vi "Shut_Down_A_Tunnel.vi"(3 "Mode":T5=enum."Run VI", 5 "Traverse line In":T2 {"Carrier_2 Q (l/min)" format="%#.2f"; "Row Duration (mins)" format="%#.1f"; "Row No" min=0; "Trace Gas Concentration (%)" min=0.0 format="%#_4f"; "Carrier_1 Q (l/min)" format="%#.4f"; "Start X" format="%#.2f"; "Start Y" format="%#.2f"; "Start Z" format="%#.2f"; "End X" format="%#.2f"; "End Y" format="%#.2f"; "End Z" format="%#.2f"; "Tunnel Speed" format="%#.2f"; "Averaging time (mins)" min=0.0 format="%#.2f"}) -> (0 "Error Message":string, 1 "Status":T1, 2 "Traverse line Out":T2 {"Carrier_2 Q (l/min)" format="%#.2f"; "Row Duration (mins)" format="%#.1f"; "Row No" min=0; "Trace Gas Concentration (%)" min=0.0 format="%#_4f"; "Carrier_1 Q (l/min)" format="%#.4f"; "Start X" format="%#.2f"; "Start Y" format="%#.2f"; "Start Z" format="%#.2f"; "End X" format="%#.2f"; "End Y" format="%#.2f"; "End Z" format="%#.2f"; "Tunnel Speed" format="%#.2f"; "Averaging time (mins)" min=0.0 format="%#.2f"})   [LabVIEW 2022 SP3]
uses:
  Gen Trav/Traverse_cluster.ctl
  Gen Trav/Spacing.ctl
  Controls/Multi_run_mode.ctl
  Controls/User_Specific_mode.ctl
  Gen Trav/Multi_Run_Status.ctl
  Controls/GMU Gas Line Name.ctl
  ADAM Client/Sub VIs/ADAM Controls/Channel_names.ctl
  ADAM Client/Sub VIs/ADAM Controls/Client_Source_Status.ctl
  ADAM Client/Sub VIs/ADAM Controls/Tunnel_speed_mode.ctl
  Globals/Trav_pos_global.vi
  Globals/Preference_global.vi
panel:
  # "X           Y          Z"
  # "Start"
  # "End"
  # "X           Y          Z"
  # "Start"
  # "End"
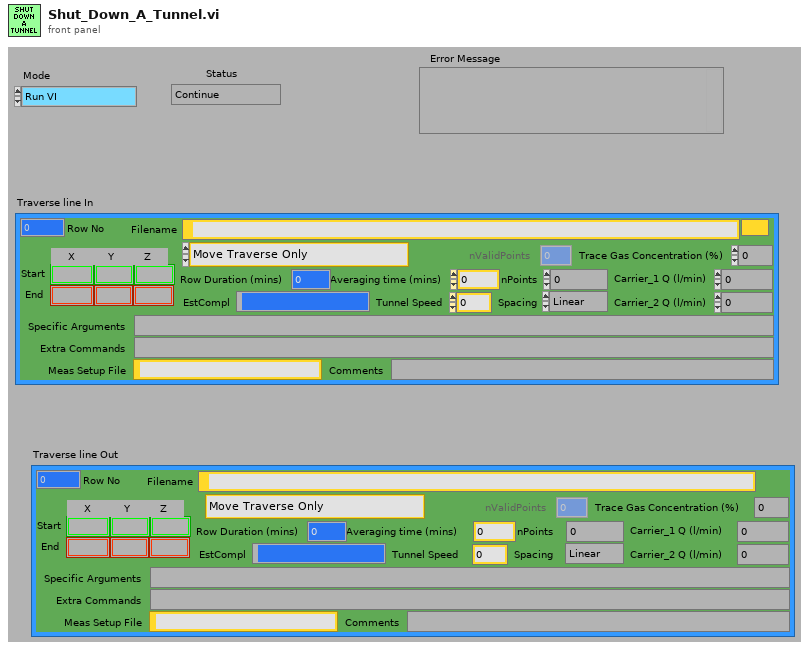
[diagram p1: front panel]
types:
  T1 = typedef "Multi_Run_Status.ctl" = enum16{"Continue", "Continue with Error", "Jump to Next Point", "Jump to Next Row", "Jump To Fall Back", "Terminate Run"}
  T2 = typedef "Traverse_cluster.ctl" = cluster{"Start X":sgl, "Start Y":sgl, "Start Z":sgl, "End X":sgl, "End Y":sgl, "End Z":sgl, "nPoints":i32, "Spacing":T3, "Filename":path, "Tunnel Speed":dbl, "Averaging time (mins)":dbl, "Extra Commands":string, "Carrier_1 Q (l/min)":dbl, "Carrier_2 Q (l/min)":dbl, "Trace Gas Concentration (%)":dbl, "Specific Arguments":string, "Comments":string, "Row No":i32, "Row Type Selector":T4, "EstCompl":string, "Row Duration (mins)":dbl, "nValidPoints":i32, "Meas Setup File":string}
  T3 = typedef "Spacing.ctl" = enum16{"Linear", "Log", "Gauss", "Specified", "N/A"}
  T4 = typedef "Multi_run_mode.ctl" = enum16{"Move Traverse Only", "Set Tunnel Speed Only", "Set Source Only", "Set Measurement Conditions", "Single Measurement", "Vertical Profile", "Lateral Profile", "Longitudinal Profile", "Multi-Axis Profile", "Explore Volume", "Auto Calibrate", "Meas Fast FID Bkgnd", "Check Beam Power", "Scanning Valve Measurement", "Run VI Named:", "Set ADAM Ch", "Wait (minutes)", "Send Message", "Synchronize With:", "Fall Back to this Row", "Turn Off Row Repeating", "Traverse 3D Volume", "Blank Row", "Jump to Fall Back Row"}
  T5 = typedef "User_Specific_mode.ctl" = enum16{"Check VI only", "Run VI"}
  T6 = typedef "GMU Gas Line Name.ctl" = enum16{"GMU1 Source", "GMU2 Source", "GMU2 Calib", "CPP GRC-A", "CPP GRC-B"}
  T7 = typedef "Channel_names.ctl" = enum16{"Active Only", "Active + Off", "All Channels", "Changeable Only", "Always Off", "Always On", "Always Off or On"}
  T8 = typedef "Client_Source_Status.ctl" = enum16{"Not Using", "Using", "Must Have"}
  T9 = typedef "Tunnel_speed_mode.ctl" = enum16{"Set Speed", "Set Speed then wait", "Is tunnel speed allowable?"}
  T10 = cluster{"second":i32, "minute":i32, "hour":i32, "day of month":i32, "month":i32, "year":i32, "day of week":i32, "day of year":i32, "is DST":i32}
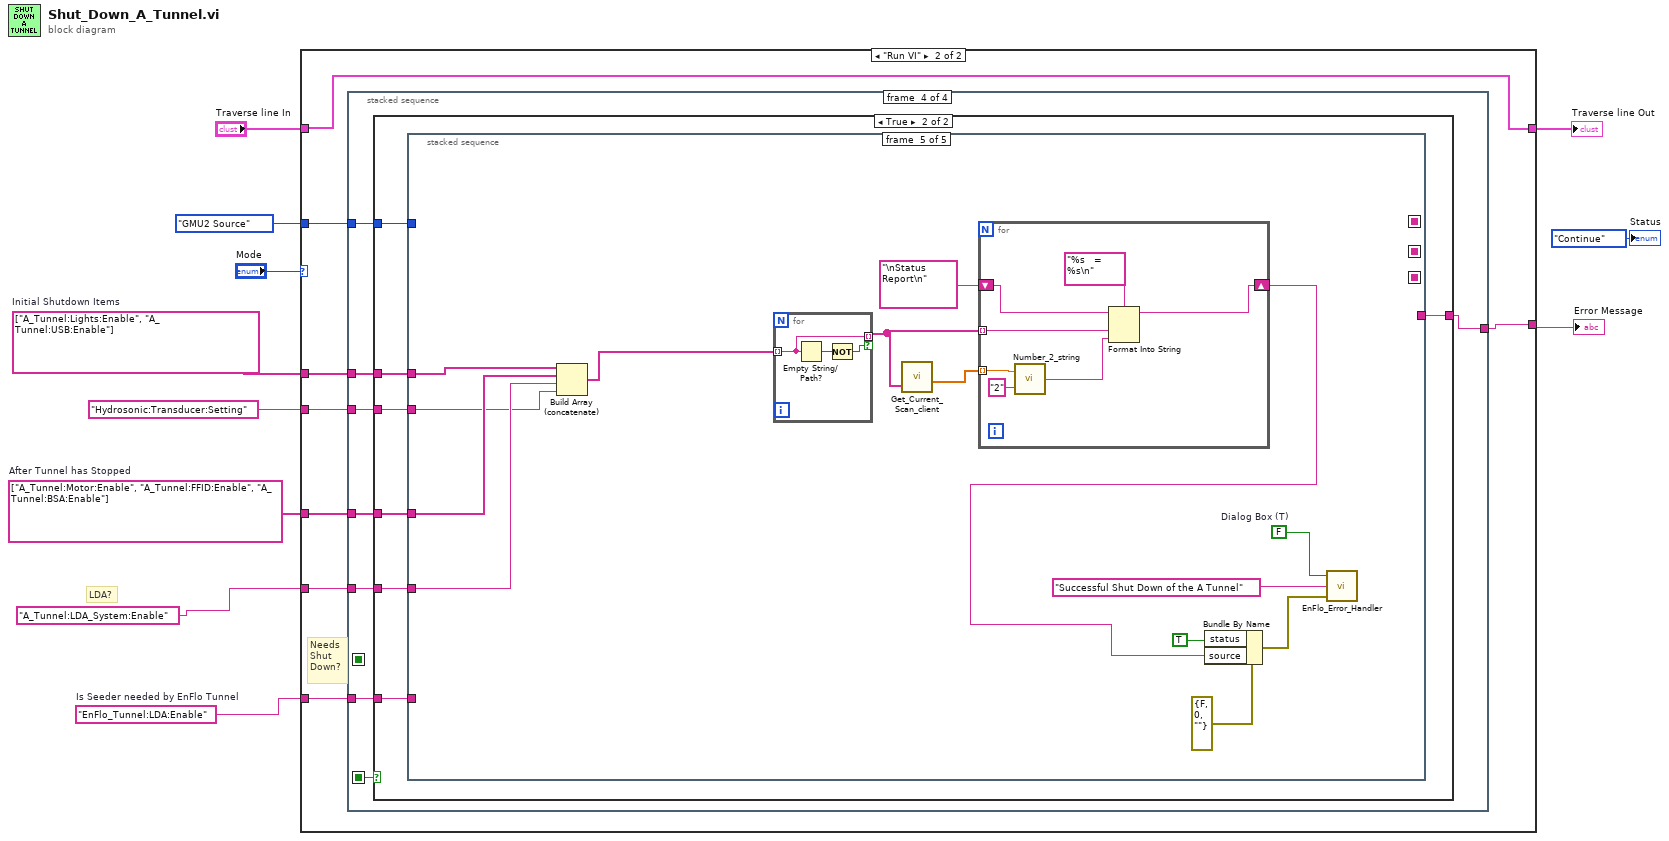
[diagram p0: block diagram]
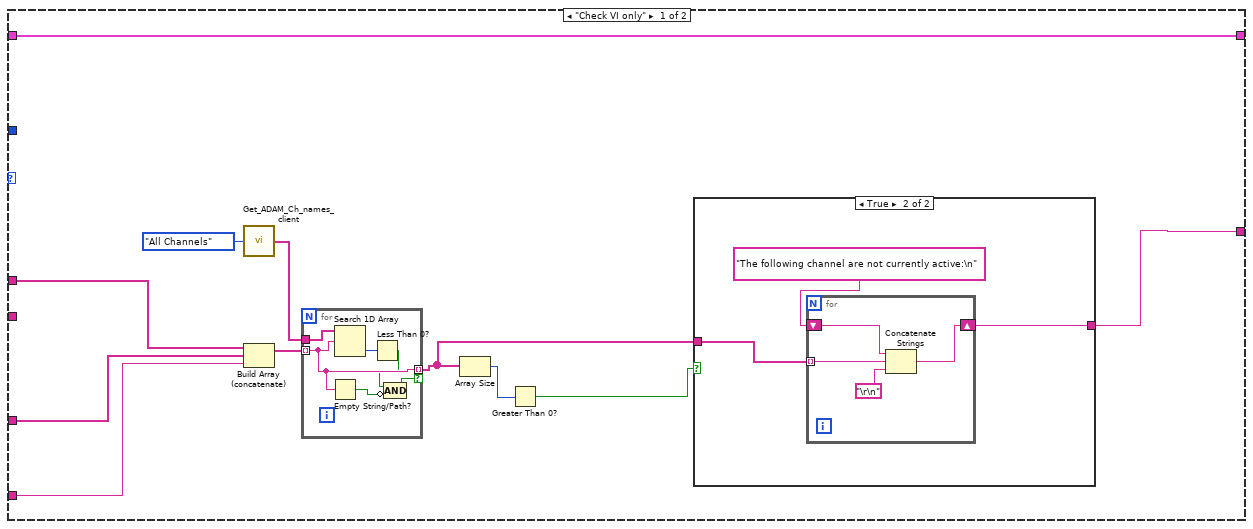
[diagram p2: hidden frame]
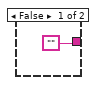
[diagram p3: hidden frame]
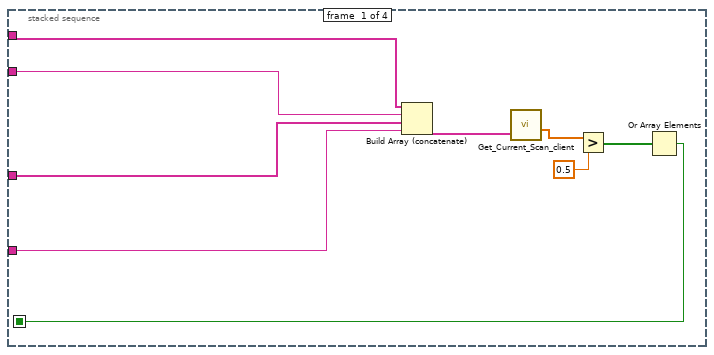
[diagram p4: hidden frame]
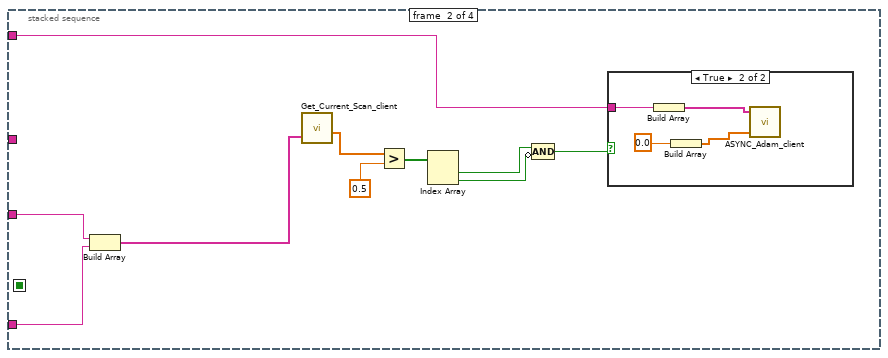
[diagram p5: hidden frame]
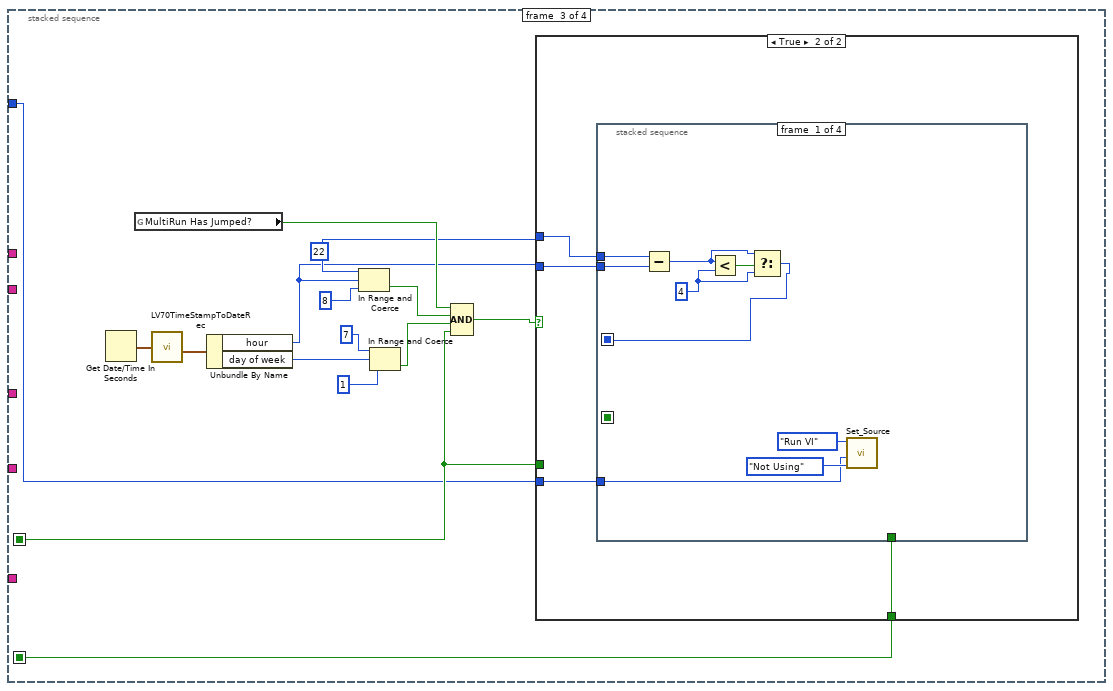
[diagram p7: hidden frame]
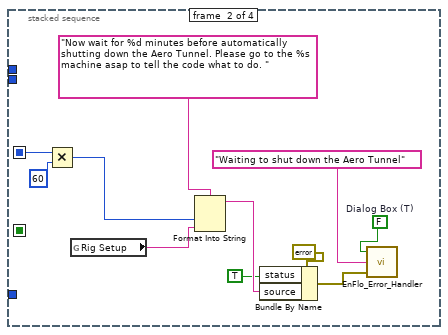
[diagram p9: hidden frame]
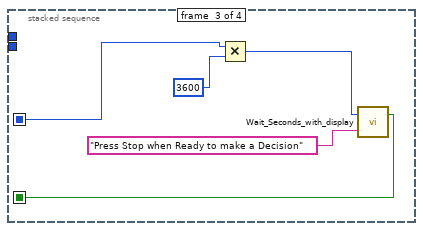
[diagram p10: hidden frame]
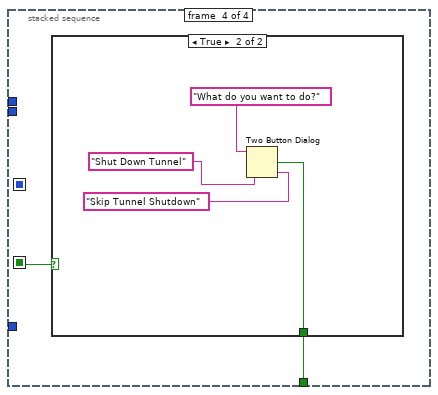
[diagram p11: hidden frame]
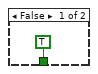
[diagram p12: hidden frame]
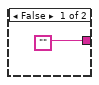
[diagram p13: hidden frame]
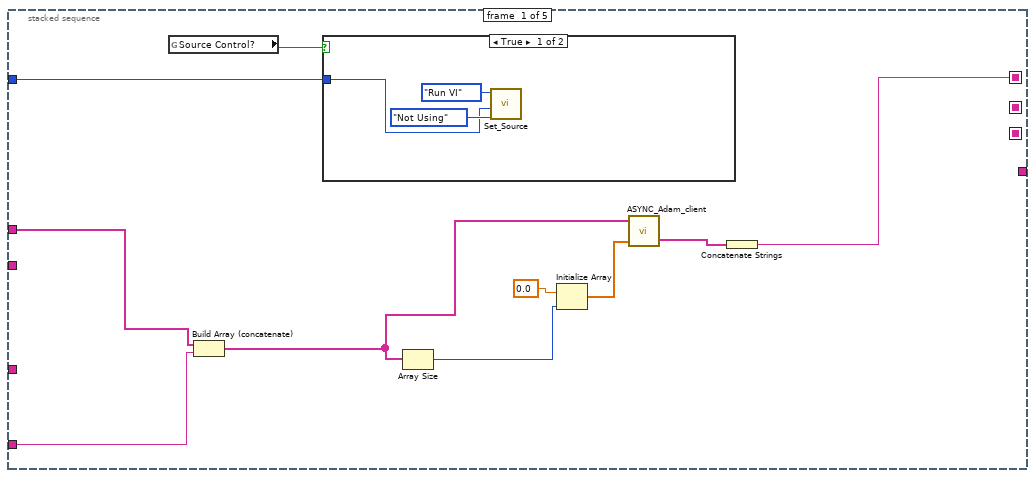
[diagram p14: hidden frame]
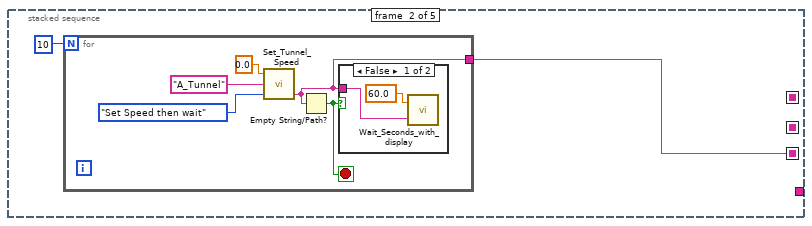
[diagram p16: hidden frame]
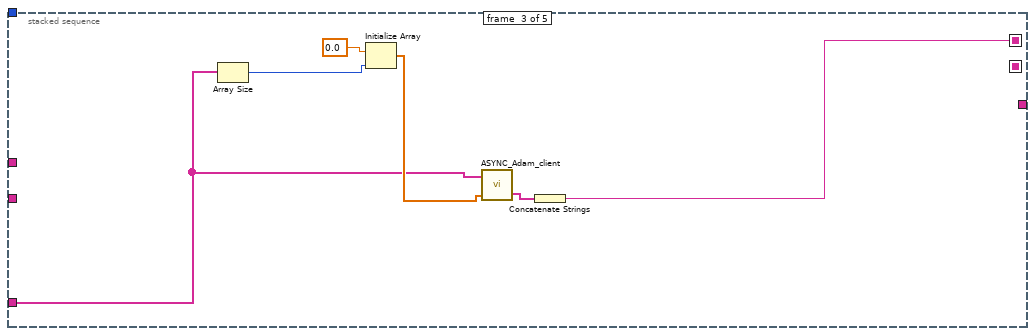
[diagram p18: hidden frame]
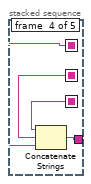
[diagram p19: hidden frame]
diagram:
  w1 = "EnFlo_Tunnel:LDA:Enable"  # Is Seeder needed by EnFlo Tunnel
  w5 = string[] ["A_Tunnel:Motor:Enable", "A_Tunnel:FFID:Enable", "A_Tunnel:BSA:Enable"]  # After Tunnel has Stopped
  w6 = string[] ["A_Tunnel:Lights:Enable", "A_Tunnel:USB:Enable"]  # Initial Shutdown Items
  # "LDA?"
  n1 = case shown="\"Run VI\"" "Mode" {
    tunnel: "Traverse line In" -> [w22 w44]
    tunnel: [w22 w44] -> w9
    tunnel: [w16 w40] -> w8
    tunnel: w6 -> [w21 w43]
    tunnel: "A_Tunnel:LDA_System:Enable" -> [w19 w42]
    tunnel: w5 -> [w20 w41]
    tunnel: w1 -> [_ w39]
    tunnel: "Hydrosonic:Transducer:Setting" -> [_ w38]
    tunnel: GMU_Gas_Line_Name."GMU2 Source" ("Gas Line Name") -> [_ w37]
    frame "Check VI only" {
      n2 = call "Get_ADAM_Ch_names_client.vi"("Channel names set"=Channel_names."All Channels") -> ("Ch names"=w15:string[])
      n3 = Build Array (concatenate)(w21, w20, w19) -> (w14:string[])
      n4 = for {
        tunnel: w15 -> [w36]
        tunnel: w14 -> [w34] mode=indexing
        tunnel: [w34] -> w17 mode=indexing if=w31
        n5 = Empty String/Path?(string/path=w34) -> (empty?=w32:bool)
        n6 = Search 1D Array(1D array=w36, element=w34) -> (index of element=w35:i32)  [unwired: 1 in]
        n7 = Less Than 0?(x=w35) -> (x < 0?=w33:bool)
        n8 = Compound Arithmetic op=AND(w33, invert w32) -> (w31:bool)
      }
      n9 = Array Size(array=w17) -> (size(s)=w12:i32)
      n10 = Greater Than 0?(x=w12) -> (x > 0?=w13:bool)
      n11 = case shown="True" w13 {
        tunnel: w17 -> [_ w26]
        tunnel: ["" w24] -> w16
        frame False {
        }
        frame True {
          n12 = for {
            tunnel: w26 -> [w29] mode=indexing
            shift-right: [w27] -> w24
            shift-left: "The following channel are not currently active:\n" -> [w28]
            n13 = Concatenate Strings(w28, w29, "\r\n") -> (w27:string)
          }
        }
      }
    }
    frame "Run VI" {
      # "Needs\nShut\nDown?"
      n14 = stacked-sequence {
        seq-local: [_ _ w70 _] -> [_ _ _ w123]
        seq-local: [w47 _ _ _] -> [_ _ w69 _]
        tunnel: w43 -> [w46 _ _ w127]
        tunnel: w42 -> [w48 w61 _ w126]
        tunnel: w41 -> [w49 _ _ w125]
        tunnel: [_ _ _ w124] -> w40
        tunnel: w39 -> [_ w60 _ w122]
        tunnel: w38 -> [w45 w62 _ w121]
        tunnel: w37 -> [_ _ w68 w120]
        frame #0 {
          n15 = Build Array (concatenate)(w46, w45, w49, w48) -> (w50:string[])
          n16 = call "Get_Current_Scan_client.vi"("multipleChannels"=w50) -> ("Numerical Values"=w51:dbl[])  [unwired: 1 in, 3 out]
          n17 = Greater?(x=w51, y=0.5) -> (0:w53:bool[])
          n18 = Or Array Elements(Boolean array=w53) -> (logical OR=w47:bool)
        }
        frame #1 {
          n19 = Build Array(w61, w60) -> (w59:string[])
          n20 = call "Get_Current_Scan_client.vi"("multipleChannels"=w59) -> ("Numerical Values"=w58:dbl[])  [unwired: 1 in, 3 out]
          n21 = Greater?(x=w58, y=0.5) -> (0:w57:bool[])
          n22 = Index Array(array=w57) -> (element #1=w56:bool, element #2=w55:bool)  [unwired: 2 in]
          n23 = Compound Arithmetic op=AND(w56, invert w55) -> (w54:bool)
          n24 = case shown="True" w54 {
            tunnel: w62 -> [_ w67]
            frame False {
            }
            frame True {
              n25 = Build Array(w67) -> (w66:string[])
              n26 = Build Array(0.0) -> (w65:dbl[])
              n27 = call "ASYNC_Adam_client.vi"("Values"=w65, "Channel Names"=w66) -> ()  [unwired: 1 in, 2 out]
            }
          }
        }
        frame #2 {
          w72 = 22 ("lower limit")
          n28 = Get Date/Time In Seconds() -> (seconds since 1Jan1904=w79:timestamp)
          n29 = global read "Trav_pos_global.vi" "MultiRun Has Jumped?"() -> (w74:bool)
          n30 = call <vilib>:"LV70TimeStampToDateRec.vi"("time stamp"=w79) -> ("date time rec"=w82:T10)
          n31 = Unbundle By Name(w82) -> ("hour"=w71:i32, "day of week"=w78:i32)
          n32 = In Range and Coerce(upper limit=w72, x=w71, lower limit=8) -> (In Range?=w75:bool)  [unwired: 1 out]
          n33 = In Range and Coerce(upper limit=7, x=w78, lower limit=1) -> (In Range?=w76:bool)  [unwired: 1 out]
          n34 = Compound Arithmetic op=AND(w74, w75, w76, w69) -> (w73:bool)
          n35 = case shown="True" w73 {
            tunnel: w72 -> [_ w87]
            tunnel: w71 -> [_ w86]
            tunnel: [w83 w85] -> w70
            tunnel: w69 -> [w83 _]
            tunnel: w68 -> [_ w84]
            frame False {
            }
            frame True {
              n36 = stacked-sequence {
                seq-local: [_ _ w109 _] -> [_ _ _ w113]
                seq-local: [w89 _ _ _] -> [_ w97 w108 _]
                tunnel: w87 -> [w96 _ _ _]
                tunnel: w86 -> [w95 _ _ _]
                tunnel: [_ _ _ w114] -> w85
                tunnel: w84 -> [w88 _ _ _]
                frame #0 {
                  w92 = 4 ("y")
                  n37 = Subtract(x=w96, y=w95) -> (x-y=w93:i32)
                  n38 = Less?(x=w93, y=w92) -> (x < y?=w94:bool)
                  n39 = Select(t=w93, s=w94, f=w92) -> (s? t:f=w89:i32)
                  n40 = call "Set_Source.vi"("Source Status"=Client_Source_Status."Not Using", "Gas Line Name"=w88, "Simulate/Run"=User_Specific_mode."Run VI") -> ()  [unwired: 2 in, 6 out]
                }
                frame #1 {
                  w100 = FALSE  # Dialog Box (T)
                  n41 = Multiply(x=w97, y=60) -> (x*y=w105:i32)
                  n42 = global read "Preference_global.vi" "Rig Setup"() -> (w106:string)
                  n43 = Format Into String(format string="Now wait for %d minutes before automatically shutting down the Aero Tunnel. Please go to the %s machine asap to tell the code what to do. ", w105, w106) -> (resulting string=w107:string)  [unwired: 2 in, 1 out]
                  n44 = Bundle By Name(cluster=errorcluster {"status"=FALSE, "code"=0, "source"=""} ("error in (no error)"), "status"=TRUE ("Bundle Element"), "source"=w107) -> (w98:errorcluster)
                  n45 = call "EnFlo_Error_Handler.vi"("error in (no error)"=w98, "Error Type"="Waiting to shut down the Aero Tunnel", "Dialog Box (F)"=w100) -> ()  [unwired: 3 out]
                }
                frame #2 {
                  n46 = Multiply(x=w108, y=3600) -> (x*y=w110:i32)
                  n47 = call "Wait_Seconds_with_display.vi"("Message"="Press Stop when Ready to make a Decision", "Seconds to wait"=w110) -> ("Stopped"=w109:bool)  [unwired: 1 out]
                }
                frame #3 {
                  n48 = case shown="True" w113 {
                    tunnel: [TRUE ("T button?") w116] -> w114
                    frame False {
                    }
                    frame True {
                      n49 = Two Button Dialog(message="What do you want to do?", 1:"Skip Tunnel Shutdown" ("F button name (\"Cancel\")"), 2:"Shut Down Tunnel" ("T button name (\"OK\")")) -> (T button?=w116:bool)
                    }
                  }
                }
              }
            }
          }
        }
        frame #3 {
          n50 = case shown="True" w123 {
            tunnel: w127 -> [_ w135]
            tunnel: w126 -> [_ w134]
            tunnel: w125 -> [_ w133]
            tunnel: ["" w132] -> w124
            tunnel: w122 -> [_ w131]
            tunnel: w121 -> [_ w130]
            tunnel: w120 -> [_ w129]
            frame False {
            }
            frame True {
              n51 = stacked-sequence {
                seq-local: [w140 _ _ _ _] -> [_ _ _ w166 _]
                seq-local: [_ _ w159 _ _] -> [_ _ _ w167 _]
                seq-local: [_ w149 _ _ _] -> [_ _ _ w164 _]
                tunnel: w135 -> [w137 _ _ _ w176]
                tunnel: w134 -> [w138 _ _ _ w178]
                tunnel: w133 -> [_ _ w158 _ w177]
                tunnel: [_ _ _ w165 _] -> w132
                tunnel: w131 -> [_ _ _ _ _]
                tunnel: w130 -> [_ _ _ _ w168]
                tunnel: w129 -> [w139 _ _ _ _]
                frame #0 {
                  n52 = global read "Trav_pos_global.vi" "Source Control?"() -> (w145:bool)
                  n53 = Build Array (concatenate)(w137, w138) -> (w136:string[])
                  n54 = case shown="True" w145 {
                    tunnel: w139 -> [w146 _]
                    frame True {
                      n55 = call "Set_Source.vi"("Source Status"=Client_Source_Status."Not Using", "Gas Line Name"=w146, "Simulate/Run"=User_Specific_mode."Run VI") -> ()  [unwired: 2 in, 6 out]
                    }
                    frame False {
                    }
                  }
                  n56 = Array Size(array=w136) -> (size(s)=w144:i32)
                  n57 = Initialize Array(0.0 ("Input Element"), w144) -> (w143:dbl[])
                  n58 = call "ASYNC_Adam_client.vi"("Values"=w143, "Channel Names"=w136) -> ("Scan Comments"=w142:string[])  [unwired: 1 in, 1 out]
                  n59 = Concatenate Strings(w142) -> (w140:string)
                }
                frame #1 {
                  n60 = for {
                    N: 10 -> [_]
                    tunnel: [w152] -> w149
                    stop <- w153 stop-if-true
                    n61 = call "Set_Tunnel_Speed.vi"("Mode"=Tunnel_speed_mode."Set Speed then wait", "Rig Name (default Empty)"="A_Tunnel", "Tunnel Velocity m/s"=0.0) -> ("Error String"=w152:string)  [unwired: 1 in, 1 out]
                    n62 = Empty String/Path?(string/path=w152) -> (empty?=w153:bool)
                    n63 = case shown="False" w153 {
                      tunnel: w152 -> [w156 _]
                      frame False {
                        n64 = call "Wait_Seconds_with_display.vi"("Message"=w156, "Seconds to wait"=60.0) -> ()  [unwired: 2 out]
                      }
                      frame True {
                      }
                    }
                  }
                }
                frame #2 {
                  n65 = Array Size(array=w158) -> (size(s)=w163:i32)
                  n66 = Initialize Array(0.0 ("Input Element"), w163) -> (w161:dbl[])
                  n67 = call "ASYNC_Adam_client.vi"("Values"=w161, "Channel Names"=w158) -> ("Scan Comments"=w160:string[])  [unwired: 1 in, 1 out]
                  n68 = Concatenate Strings(w160) -> (w159:string)
                }
                frame #3 {
                  n69 = Concatenate Strings(w164, w167, w166) -> (w165:string)
                }
                frame #4 {
                  w174 = FALSE  # Dialog Box (T)
                  n70 = Build Array (concatenate)(w176, w177, w178, w168) -> (w169:string[])
                  n71 = for {
                    tunnel: w169 -> [w182] mode=indexing
                    tunnel: [w182] -> w175 mode=indexing if=w183
                    n72 = Empty String/Path?(string/path=w182) -> (empty?=w184:bool)
                    n73 = Not(x=w184) -> (.not. x?=w183:bool)
                  }
                  n74 = call "Get_Current_Scan_client.vi"("multipleChannels"=w175) -> ("Numerical Values"=w179:dbl[])  [unwired: 1 in, 3 out]
                  n75 = for {
                    tunnel: w175 -> [w191] mode=indexing
                    shift-right: [w188] -> w180
                    shift-left: "\nStatus Report\n" -> [w189]
                    tunnel: w179 -> [w187] mode=indexing
                    n76 = call "Number_2_string.vi"("precision"="2", "number"=w187) -> ("String"=w185:string)
                    n77 = Format Into String(format string="%s   =  %s\n", initial string=w189, w191, w185) -> (resulting string=w188:string)  [unwired: 1 in, 1 out]
                  }
                  n78 = Bundle By Name(cluster=errorcluster {"status"=FALSE, "code"=0, "source"=""} ("error in (no error)"), "status"=TRUE ("Bundle Element"), "source"=w180) -> (w173:errorcluster)
                  n79 = call "EnFlo_Error_Handler.vi"("error in (no error)"=w173, "Error Type"="Successful Shut Down of the A Tunnel", "Dialog Box (F)"=w174) -> ()  [unwired: 3 out]
                }
              }
            }
          }
        }
      }
    }
  }
  "Traverse line Out" <- w9
  "Error Message" <- w8
  "Status" <- Multi_Run_Status."Continue" ("Status")
